vi "ConvertHandle.vi"(2 "Camera Reference In":i64, 3 "QT Ref In":T1) -> (0 "QT Ref Out":T1, 1 "Camera Reference":i64)   [LabVIEW 2022 SP3]
uses:
  <vilib>/addons/RoboLab/ImageProcessing/QTLIB_2595_LV86/QT_Ref.ctl
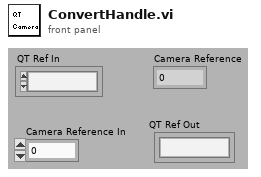
[diagram p1: front panel]
types:
  T1 = typedef "QT_Ref.ctl" = refnum<k1>
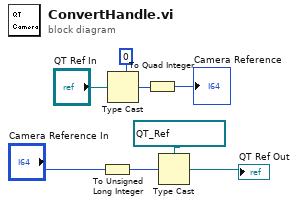
[diagram p0: block diagram]
diagram:
  w3 = T1 refnum items=["QT refnum"] ("QT Ref Out")
  n1 = To Unsigned Long Integer(number="Camera Reference In") -> (unsigned 32bit integer=w4:u32)
  n2 = Type Cast(type=u32 0, x="QT Ref In") -> (*(type *) &x=w7:u32)
  n3 = To Quad Integer(1:w7) -> (0:→"Camera Reference":i64)
  n4 = Type Cast(type=w3, x=w4) -> (*(type *) &x=→"QT Ref Out":T1)
